vi "AKD Create MT.vi"(0 "TCP Refnum in":refnum<k5>, 5 "Motion Task parameters":T1, 7 "Task no":u16, 9 "Next MT?":bool, 11 "error in":errorcluster, 12 "Motion type":enum16{"Rel", "Abs"}(ring)=enum."Abs") -> (4 "TCP Refnum out":refnum<k5>, 15 "error out":errorcluster)   [LabVIEW 2019]
doc: "This VI will define a new motion task in the AKD drive with the paramters of position, velocity, motion type, acceleration, deceleration and whether to immediately run a subsequent MT.\nThe motion type will always be set to type 2 (relative motion). Once a MT has been defined it can be initiated using AKD Move.vi"
uses:
  MODBUS/NI Modbus.llb/MB Ethernet Master Query Write Multiple Registers (poly).vi
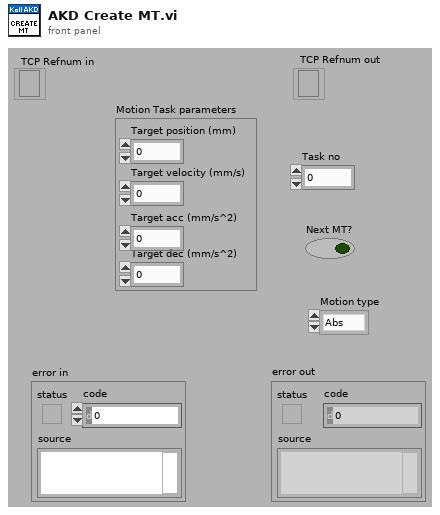
[diagram p1: front panel]
types:
  T1 = cluster{"Target position (mm)":sgl, "Target velocity (mm/s)":sgl, "Target acc (mm/s^2)":sgl, "Target dec (mm/s^2)":sgl}
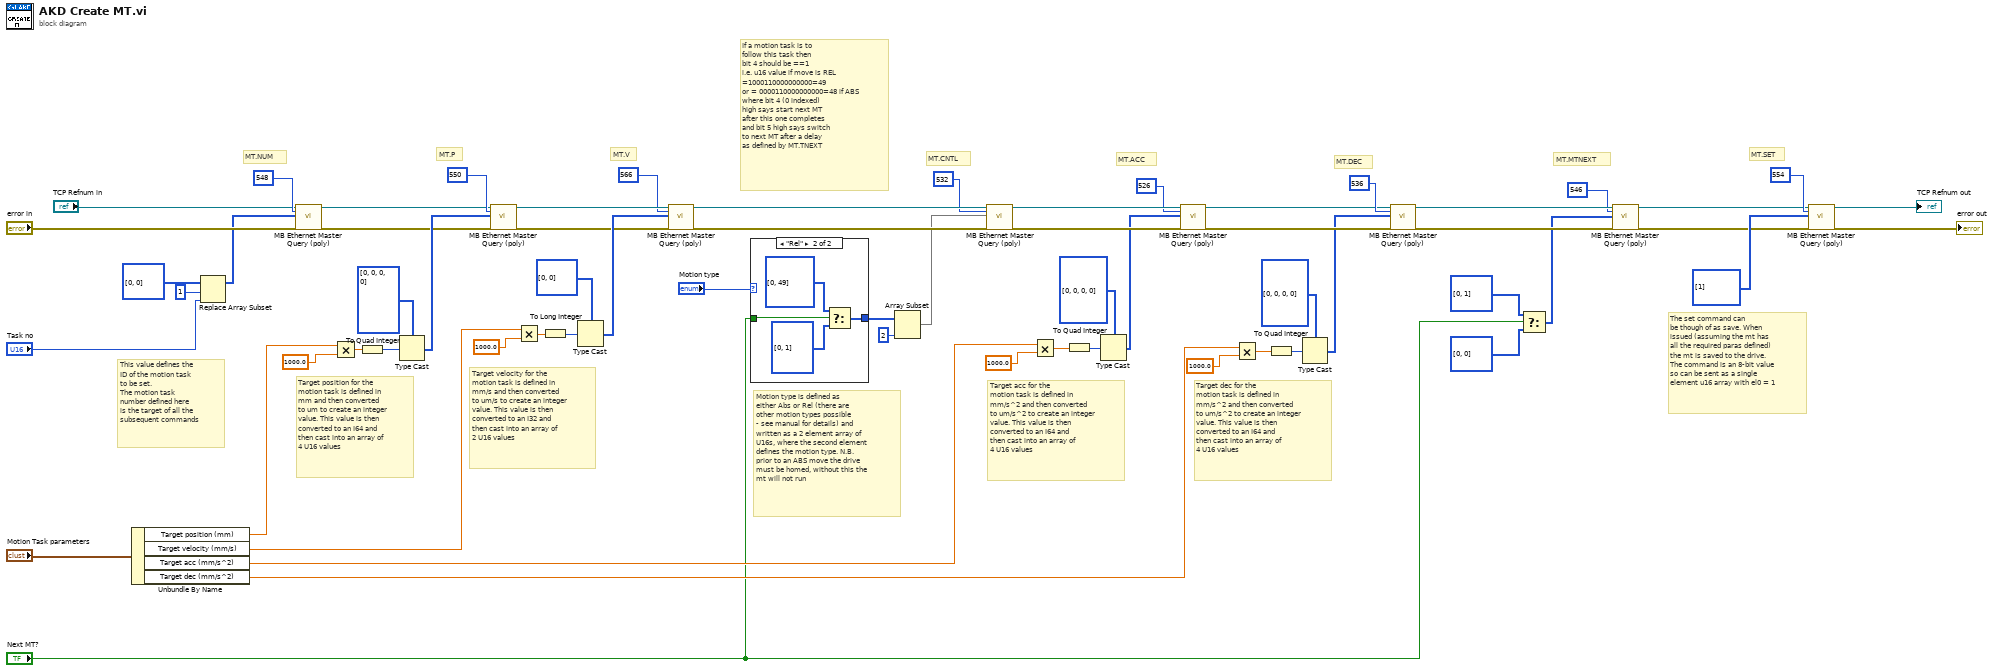
[diagram p0: block diagram]
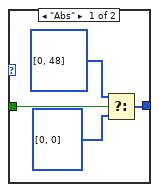
[diagram p2: hidden frame]
diagram:
  # "If a motion task is to\nfollow this task then \nbit 4 should be ==1\ni.e. u16 value if move is REL \n=1000110000000000=49\nor = 0000110000000000=48 if ABS\nwhere bit 4 (0 indexed)\nhigh says start next MT \nafter this one completes\nand bit 5 high says switch\nto next MT after a delay\nas defined by MT.TNEXT"
  # "MT.MTNEXT"
  # "The set command can\nbe though of as save. When\nissued (assuming the mt has \nall the required paras defined)\nthe mt is saved to the drive.\nThe command is an 8-bit value\nso can be sent as a single\nelement u16 array with el0 = 1"
  # "Target dec for the\nmotion task is defined in\nmm/s^2 and then converted\nto um/s^2 to create an integer\nvalue. This value is then\nconverted to an I64 and\nthen cast into an array of \n4 U16 values"
  # "Target acc for the\nmotion task is defined in\nmm/s^2 and then converted\nto um/s^2 to create an integer\nvalue. This value is then\nconverted to an I64 and\nthen cast into an array of \n4 U16 values"
  # "Motion type is defined as\neither Abs or Rel (there are\nother motion types possible\n- see manual for details) and\nwritten as a 2 element array of\nU16s, where the second element\ndefines the motion type. N.B.\nprior to an ABS move the drive\nmust be homed, without this the\nmt will not run"
  # "Target velocity for the\nmotion task is defined in\nmm/s and then converted\nto um/s to create an integer\nvalue. This value is then\nconverted to an I32 and\nthen cast into an array of \n2 U16 values"
  # "Target position for the\nmotion task is defined in\nmm and then converted\nto um to create an integer\nvalue. This value is then\nconverted to an I64 and\nthen cast into an array of \n4 U16 values"
  # "This value defines the \nID of the motion task\nto be set.\nThe motion task\nnumber defined here\nis the target of all the \nsubsequent commands"
  # "MT.DEC"
  # "MT.ACC"
  # "MT.SET"
  # "MT.CNTL"
  # "MT.V"
  # "MT.P"
  # "MT.NUM"
  n1 = Unbundle By Name("Motion Task parameters") -> ("Target position (mm)"=w21:sgl, "Target velocity (mm/s)"=w20:sgl, "Target acc (mm/s^2)"=w19:sgl, "Target dec (mm/s^2)"=w18:sgl)
  n2 = Replace Array Subset(array=u16[] [0, 0], new element="Task no", index=1) -> (w12:u16[])
  n3 = call-poly "MB Ethernet Master Query (poly).vi"("TCP Connection Refnum in"="TCP Refnum in", "Starting Address"=u16 548, "Registers"=w12, "error in"="error in") -> ("TCP Connection Refnum (dup)"=w35:refnum<k5>, "error out"=w34:errorcluster)  [unwired: 13 in, 1 out]
  n4 = Multiply(x=w21, y=sgl 1000.0) -> (x*y=w33:sgl)
  n5 = To Quad Integer(1:w33) -> (0:w31:i64)
  n6 = Type Cast(type=u16[] [0, 0, 0, 0], x=w31) -> (*(type *) &x=w61:u16[])
  n7 = call-poly "MB Ethernet Master Query (poly).vi"("TCP Connection Refnum in"=w35, "Starting Address"=u16 550, "Registers"=w61, "error in"=w34) -> ("TCP Connection Refnum (dup)"=w58:refnum<k5>, "error out"=w51:errorcluster)  [unwired: 13 in, 1 out]
  n8 = Multiply(x=w20, y=sgl 1000.0) -> (x*y=w29:sgl)
  n9 = To Long Integer(number=w29) -> (32bit integer=w30:i32)
  n10 = Type Cast(type=u16[] [0, 0], x=w30) -> (*(type *) &x=w59:u16[])
  n11 = call-poly "MB Ethernet Master Query (poly).vi"("TCP Connection Refnum in"=w58, "Starting Address"=u16 566, "Registers"=w59, "error in"=w51) -> ("TCP Connection Refnum (dup)"=w56:refnum<k5>, "error out"=w50:errorcluster)  [unwired: 13 in, 1 out]
  n12 = case shown="\"Rel\"" "Motion type" {
    tunnel: [w67 w72] -> w52
    tunnel: "Next MT?" -> [w68 w71]
    frame "Abs" {
      n13 = Select(t=u16[] [0, 48], s=w68, f=u16[] [0, 0]) -> (s? t:f=w67:u16[])
    }
    frame "Rel" {
      n14 = Select(t=u16[] [0, 49], s=w71, f=u16[] [0, 1]) -> (s? t:f=w72:u16[])
    }
  }
  n15 = Array Subset(array=w52, length=2) -> (w1:u16[])  [unwired: 1 in]
  n16 = call-poly "MB Ethernet Master Query (poly).vi"("TCP Connection Refnum in"=w56, "Starting Address"=u16 532, "Registers"=w1, "error in"=w50) -> ("TCP Connection Refnum (dup)"=w48:refnum<k5>, "error out"=w43:errorcluster)  [unwired: 13 in, 1 out]
  n17 = Multiply(x=w19, y=sgl 1000.0) -> (x*y=w39:sgl)
  n18 = To Quad Integer(1:w39) -> (0:w38:i64)
  n19 = Type Cast(type=u16[] [0, 0, 0, 0], x=w38) -> (*(type *) &x=w42:u16[])
  n20 = call-poly "MB Ethernet Master Query (poly).vi"("TCP Connection Refnum in"=w48, "Starting Address"=u16 526, "Registers"=w42, "error in"=w43) -> ("TCP Connection Refnum (dup)"=w41:refnum<k5>, "error out"=w44:errorcluster)  [unwired: 13 in, 1 out]
  n21 = Multiply(x=w18, y=sgl 1000.0) -> (x*y=w26:sgl)
  n22 = To Quad Integer(1:w26) -> (0:w27:i64)
  n23 = Type Cast(type=u16[] [0, 0, 0, 0], x=w27) -> (*(type *) &x=w23:u16[])
  n24 = call-poly "MB Ethernet Master Query (poly).vi"("TCP Connection Refnum in"=w41, "Starting Address"=u16 536, "Registers"=w23, "error in"=w44) -> ("TCP Connection Refnum (dup)"=w8:refnum<k5>, "error out"=w9:errorcluster)  [unwired: 13 in, 1 out]
  n25 = Select(t=u16[] [0, 1] ("Registers"), s="Next MT?", f=u16[] [0, 0] ("Registers")) -> (s? t:f=w4:u16[])
  n26 = call-poly "MB Ethernet Master Query (poly).vi"("TCP Connection Refnum in"=w8, "Starting Address"=u16 546, "Registers"=w4, "error in"=w9) -> ("TCP Connection Refnum (dup)"=w11:refnum<k5>, "error out"=w10:errorcluster)  [unwired: 13 in, 1 out]
  n27 = call-poly "MB Ethernet Master Query (poly).vi"("TCP Connection Refnum in"=w11, "Starting Address"=u16 554, "Registers"=u16[] [1], "error in"=w10) -> ("TCP Connection Refnum (dup)"=→"TCP Refnum out":refnum<k5>, "error out"=→"error out":errorcluster)  [unwired: 13 in, 1 out]
